vi "testProcessPacket.vi"(8 "error in (no error)":errorcluster) -> (0 "error out":errorcluster)   [LabVIEW 2018]
doc: "Test the processPacket subVI."
uses:
  <vilib>/addons/_JKI Toolkits/Caraya/classes/Test/Test.lvclass
  <vilib>/addons/_JKI Toolkits/Caraya/classes/Assert/Assert.lvclass
  src/TcpServer/TcpServer.lvclass
  src/TcpServer/typedef/tcpPacketTypeDef.ctl
  <vilib>/addons/_JKI Toolkits/Caraya/classes/Assert/Assert Equal Value_Variant.vi
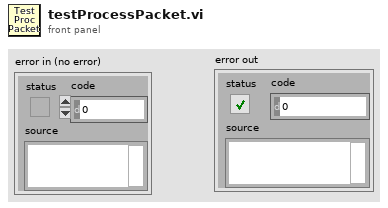
[diagram p1: front panel]
types:
  T1 = typedef "TcpServer.lvclass/tcpPacketTypeDef.ctl" = cluster{"packet":string, "firstPacket":bool, "firstConnection":bool}
  T2 = typedef "TcpServer.lvclass/packetConnIDTypeDef.ctl" = cluster{"packet":string, "firstPacket":bool, "firstConnection":bool}
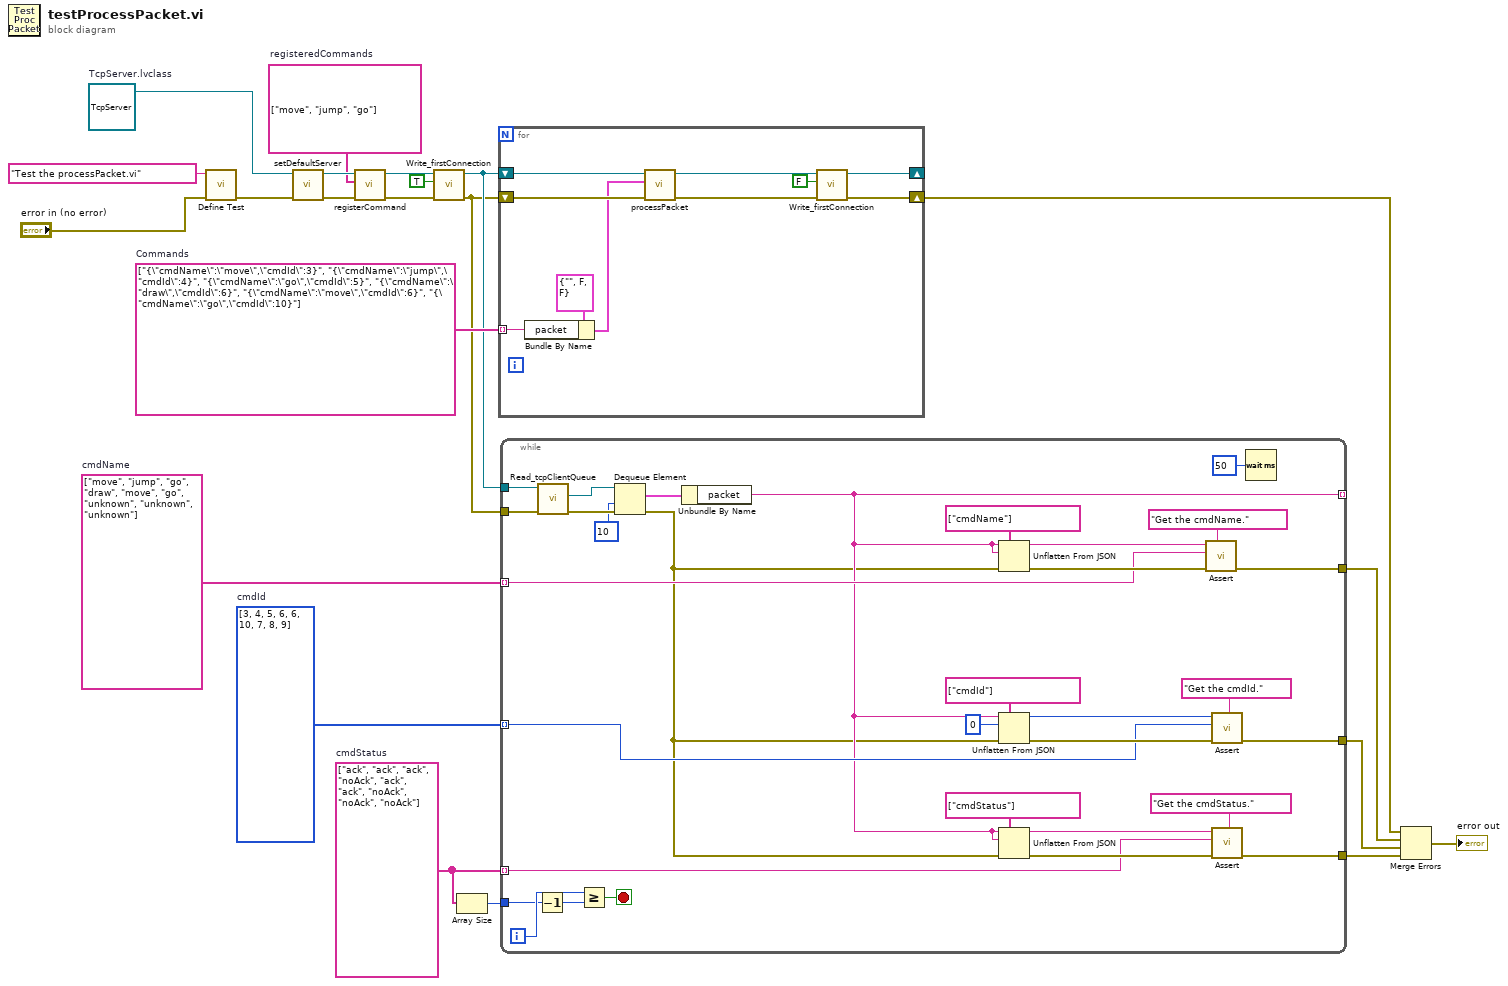
[diagram p0: block diagram]
diagram:
  w3 = string[] ["ack", "ack", "ack", "noAck", "ack", "ack", "noAck", "noAck", "noAck"]  # cmdStatus
  w7 = i32[] [3, 4, 5, 6, 6, 10, 7, 8, 9]  # cmdId
  w8 = string[] ["move", "jump", "go", "draw", "move", "go", "unknown", "unknown", "unknown"]  # cmdName
  w14 = string[] ["{\"cmdName\":\"move\",\"cmdId\":3}", "{\"cmdName\":\"jump\",\"cmdId\":4}", "{\"cmdName\":\"go\",\"cmdId\":5}", "{\"cmdName\":\"draw\",\"cmdId\":6}", "{\"cmdName\":\"move\",\"cmdId\":6}", "{\"cmdName\":\"go\",\"cmdId\":10}"]  # Commands
  w15 = string[] ["move", "jump", "go"]  # registeredCommands
  w19 = refnum<class "TcpServer.lvclass"> refnum  # TcpServer.lvclass
  n1 = call <vilib>:"Define Test.vi"("error in (no error)"="error in (no error)", "Label (VI Title)"="Test the processPacket.vi") -> ("error out"=w21:errorcluster)  [unwired: 9 in]
  n2 = call "setDefaultServer.vi"("error in (no error)"=w21, "TcpServer.lvclass"=w19) -> ("error out"=w17:errorcluster, "tcpServer out"=w16:refnum<class "TcpServer.lvclass">)  [unwired: 8 in]
  n3 = call "registerCommand.vi"("error in (no error)"=w17, "registeredCommands"=w15, "tcpServer in"=w16) -> ("error out"=w18:errorcluster, "tcpServer out"=w13:refnum<class "TcpServer.lvclass">)  [unwired: 7 in]
  n4 = call "Write_firstConnection.vi"("error in (no error)"=w18, "firstConnection"=TRUE, "TcpServer in"=w13) -> ("error out"=w9:errorcluster, "TcpServer out"=w10:refnum<class "TcpServer.lvclass">)  [unwired: 7 in]
  n5 = Array Size(array=w3) -> (size(s)=w2:i32)
  n6 = for {
    tunnel: w14 -> [w28] mode=indexing
    shift-right: [w24] -> _
    shift-left: w10 -> [w30]
    shift-right: [w26] -> w1
    shift-left: w9 -> [w32]
    n7 = Bundle By Name(cluster=T1 {"packet"="", "firstPacket"=FALSE, "firstConnection"=FALSE} ("packetConnID"), "packet"=w28) -> (w29:T1)
    n8 = call "processPacket.vi"("error in (no error)"=w32, "tcpPacket"=w29, "tcpServer in"=w30) -> ("error out"=w27:errorcluster, "tcpServer out"=w25:refnum<class "TcpServer.lvclass">)  [unwired: 7 in]
    n9 = call "Write_firstConnection.vi"("error in (no error)"=w27, "firstConnection"=FALSE, "TcpServer in"=w25) -> ("error out"=w26:errorcluster, "TcpServer out"=w24:refnum<class "TcpServer.lvclass">)  [unwired: 7 in]
  }
  n10 = while {
    tunnel: w10 -> [w61]
    tunnel: w9 -> [w60]
    tunnel: w8 -> [w50] mode=indexing
    tunnel: w7 -> [w44] mode=indexing
    tunnel: w3 -> [w43] mode=indexing
    tunnel: [w42] -> w6
    tunnel: [w41] -> w5
    tunnel: [w40] -> w4
    tunnel: [w39] -> _ mode=indexing
    tunnel: w2 -> [w35]
    i -> [w36]
    stop <- w37 stop-if-true
    n11 = Decrement(x=w35) -> (x-1=w34:i32)
    n12 = call "Read_tcpClientQueue.vi"("error in (no error)"=w60, "tcpServer in"=w61) -> ("error out"=w63:errorcluster, "tcpClientQueue"=w62:refnum<queue>)  [unwired: 7 in, 1 out]
    n13 = Greater Or Equal?(x=w36, y=w34) -> (x >= y?=w37:bool)
    n14 = Dequeue Element(queue=w62, timeout in ms (-1)=10, error in (no error)=w63) -> (element=w64:T2, error out=w33:errorcluster)  [unwired: 2 out]
    n15 = Unbundle By Name(w64) -> ("packet"=w39:string)
    n16 = Unflatten From JSON(path=string[] ["cmdName"], JSON string=w39, type and defaults=w39, error in (no error)=w33) -> (value=w57:string, error out=w54:errorcluster)  [unwired: 3 in]
    n17 = Unflatten From JSON(path=string[] ["cmdId"], JSON string=w39, type and defaults=0, error in (no error)=w33) -> (value=w58:i32, error out=w53:errorcluster)  [unwired: 3 in]
    n18 = Unflatten From JSON(path=string[] ["cmdStatus"], JSON string=w39, type and defaults=w39, error in (no error)=w33) -> (value=w46:string, error out=w48:errorcluster)  [unwired: 3 in]
    n19 = call-poly <vilib>:"Assert.vi"("Label"="Get the cmdName.", "error in (no error)"=w54, "Y"=w50, "X"=w57) -> ("error out"=w40:errorcluster)  [unwired: 7 in]
    n20 = call-poly <vilib>:"Assert.vi"("Label"="Get the cmdId.", "error in (no error)"=w53, "Y"=w44, "X"=w58) -> ("error out"=w41:errorcluster)  [unwired: 7 in]
    n21 = call-poly <vilib>:"Assert.vi"("Label"="Get the cmdStatus.", "error in (no error)"=w48, "Y"=w43, "X"=w46) -> ("error out"=w42:errorcluster)  [unwired: 7 in]
    n22 = Wait (ms)(milliseconds to wait=u32 50) -> ()  [unwired: 1 out]
  }
  n23 = Merge Errors(w1, w4, w5, w6) -> (→"error out":errorcluster)
